vi "Teleop.vi"(10 "Match Info":T2={"Autonomous Elapsed Seconds"=0.0, "TeleOp Elapsed Seconds"=0.0, "Disabled Elapsed Seconds"=0.0, "Visited Autonomous"=FALSE, "Visited TeleOp"=FALSE, "Visited Disabled"=FALSE, "Autonomous Settings"={"Autonomous Style"=enum."Independent", "VI Refnum"=refnum}}, 11 "Call Context":T3) -> ()   [LabVIEW 2023]
doc: "This VI is called for each TeleOp packet received from the DS where the robot is not disabled. It is often used to read from the joysticks and update I/O or to update setpoints for timed control loops. It should complete and return within 20 milliseconds or it may miss DS packets."
uses:
  <vilib>/Rock Robotics/WPI/DriverStation/WPI_DriverStationDerivedRobotMode.ctl
  <vilib>/Rock Robotics/WPI/DriverStation/WPI_DriverStationMatch Info.ctl
  <vilib>/Rock Robotics/WPI/Solenoid/WPI_SolenoidValue.ctl
  <vilib>/Rock Robotics/WPI/ThirdParty/REV Robotics/REVLib/Typedef/Spark MAX Control Type.ctl
  <vilib>/Rock Robotics/Network Tables/NT Read Boolean.vi
  <vilib>/Rock Robotics/Network Tables/NT Read Number.vi
  <vilib>/Rock Robotics/WPI/Solenoid/WPI_SolenoidSetEnum.vi
  <vilib>/Rock Robotics/WPI/Solenoid/WPI_SolenoidGetEnum.vi
panel:
  in  "FIRE!":bool
  in  "spin up SHOOTER":bool
  in  "set motors to ZERO":bool
  out "NOTE DIO":bool
  out "Hard Limit Fwd 2":bool
  out "Hard Limit Rev 2":bool
  out "Hard Limit Fwd":bool
  out "Hard Limit Rev":bool
  out "Value 2":T1
  out "Value":T1
  in  "LOCK?":bool=TRUE
  in  "FLAP?":bool=TRUE
  in  "RIGHT":dbl(slide) scale=-1.0..1.0
  in  "LEFT":dbl(slide) scale=-1.0..1.0
  in  "SHOOTER":dbl(slide) scale=-1.0..1.0
  in  "INTAKE":dbl(slide) scale=-1.0..1.0
  in  "LOADER":dbl(slide) scale=-1.0..1.0
  out "Sample Slider 0":dbl(slide) scale=0.0..5.0
  out "Sample Boolean 1":bool
  out "Sample Boolean 0":bool
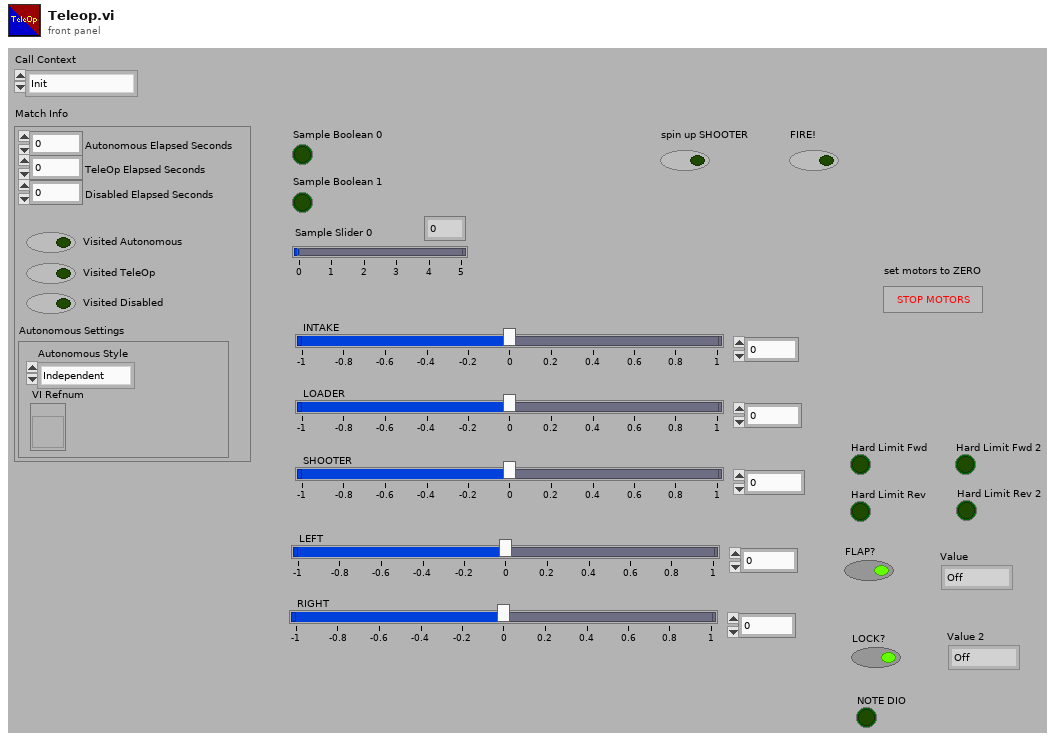
[diagram p1: front panel]
types:
  T1 = typedef "WPI_SolenoidValue.ctl" = enum16{"Off", "On", "Forward", "Reverse"}
  T2 = typedef "WPI_DriverStationMatch Info.ctl" = cluster{"Autonomous Elapsed Seconds":dbl, "TeleOp Elapsed Seconds":dbl, "Disabled Elapsed Seconds":dbl, "Visited Autonomous":bool, "Visited TeleOp":bool, "Visited Disabled":bool, "Autonomous Settings":cluster{"Autonomous Style":enum16{"Iterative", "Independent"}, "VI Refnum":refnum<vi>}}
  T3 = typedef "WPI_DriverStationDerivedRobotMode.ctl" = enum16{"Init", "Execute", "Stop"}
  T4 = typedef "Spark MAX Control Type.ctl" = enum16{"Percent VBus", "Voltage", "Velocity", "Position", "Smart Motion", "Current", "Smart Velocity"}
  T5 = typedef "WPI_MotorControlDeviceRef.ctl" = cluster{"DeviceStatus":errorcluster, "Type":T6, "PWM":cluster{"PWM Channel":T7, "DeadBand":T8}, "CAN":cluster{"Device Number":u8, "SetOutput VI Ref":variant, "GetOutput VI Ref":variant, "Enable VI Ref":variant, "Disable VI Ref":variant, "Data":variant}, "Invert":bool, "DIO PWM":cluster{"PWM \"Enable\" Channel":T7, "DIOChannel":T9, "PWM Rate":dbl}}
  T6 = typedef "WPI_MotorControlType.ctl" = enum16{"PWM", "CAN", "DIO PWM"}
  T7 = typedef "FPGA_DIOPWMChannel.ctl" = enum8{"PWM 0", "PWM 1", "PWM 2", "PWM 3", "PWM 4", "PWM 5", "PWM 6", "PWM 7", "PWM 8", "PWM 9", "PWM MXP 0", "PWM MXP 1", "PWM MXP 2", "PWM MXP 3", "PWM MXP 4", "PWM MXP 5", "PWM MXP 6", "PWM MXP 7", "PWM MXP 8", "PWM MXP 9", "Invalid"}
  T8 = typedef "WPI_PWMDeadband.ctl" = cluster{"Name":string, "maxPositivePwm":i32, "minPositivePwm":i32, "centerPwm":i32, "maxNegativePwm":i32, "minNegativePwm":i32, "angularRange":u16}
  T9 = typedef "FPGA_DIOChannel.ctl" = enum8{"DIO 0", "DIO 1", "DIO 2", "DIO 3", "DIO 4", "DIO 5", "DIO 6", "DIO 7", "DIO 8", "DIO 9", "DIO MXP 0", "DIO MXP 1", "DIO MXP 2", "DIO MXP 3", "DIO MXP 4", "DIO MXP 5", "DIO MXP 6", "DIO MXP 7", "DIO MXP 8", "DIO MXP 9", "DIO MXP 10", "DIO MXP 11", "DIO MXP 12", "DIO MXP 13", "DIO MXP 14", "DIO MXP 15", "SPI Port CS1", "SPI Port CS2", "SPI Port CS3", "SPI Port MISO", "SPI Port MOSI", "Invalid"}
  T10 = typedef "WPI_SolenoidDevRef.ctl" = cluster{"DevStatus":errorcluster, "Pneumatics Control Module":u8, "Forward Solenoid Channel":T11, "Reverse Solenoid Channel":T11}
  T11 = typedef "WPI_SolenoidChannel.ctl" = enum8{"Solenoid 0", "Solenoid 1", "Solenoid 2", "Solenoid 3", "Solenoid 4", "Solenoid 5", "Solenoid 6", "Solenoid 7", "Solenoid 8", "Solenoid 9", "Solenoid 10", "Solenoid 11", "Solenoid 12", "Solenoid 13", "Solenoid 14", "Solenoid 15", "Invalid"}
  T12 = typedef "WPI_DigitalInputDevRef.ctl" = cluster{"DevStatus":errorcluster, "DIO Channel":T9}
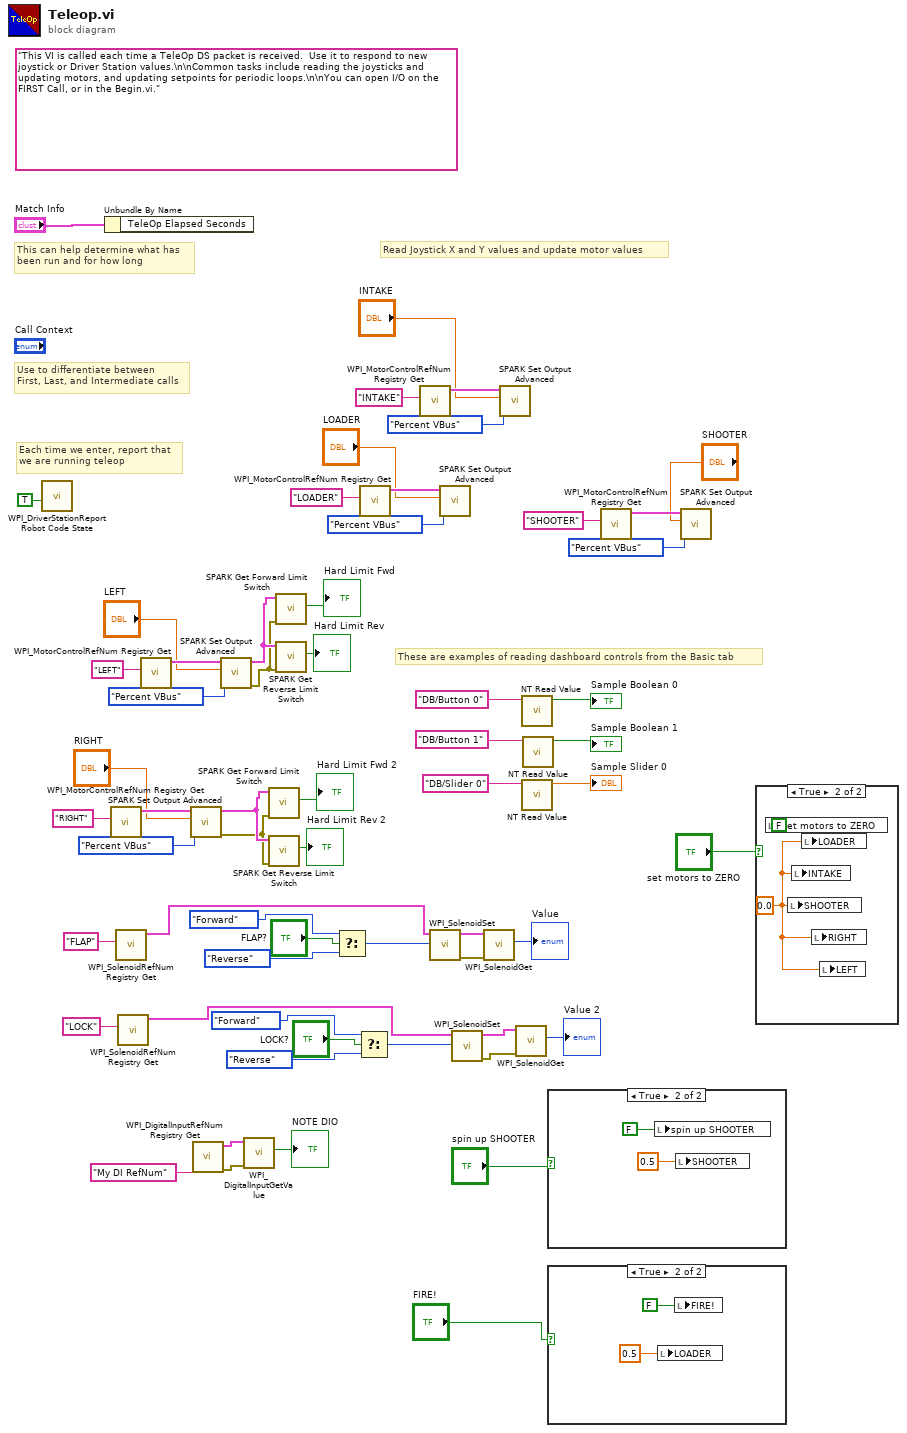
[diagram p0: block diagram]
diagram:
  (unwired) "This VI is called each time a TeleOp DS packet is received.  Use it to respond to new joystick or Driver Station values.\n\nCommon tasks include reading the joysticks and updating motors, and updating setpoints for periodic loops.\n\nYou can open I/O on the FIRST Call, or in the Begin.vi."
  # "These are examples of reading dashboard controls from the Basic tab"
  # "Each time we enter, report that\nwe are running teleop"
  # "Use to differentiate between\nFirst, Last, and Intermediate calls"
  # "This can help determine what has\nbeen run and for how long"
  # "Read Joystick X and Y values and update motor values"
  n1 = call <vilib>:"WPI_DriverStationReport Robot Code State.vi"("TeleOp"=TRUE ("Autonomous")) -> ()  [unwired: 10 in, 1 out]
  n2 = Unbundle By Name("Match Info") -> ()  [unwired: 1 out]
  n3 = call <vilib>:"WPI_MotorControlRefNum Registry Get.vi"("refnum name"="RIGHT") -> ("MotorControlDevRef"=w37:T5)  [unwired: 9 in, 1 out]
  n4 = call <vilib>:"WPI_SolenoidRefNum Registry Get.vi"("refnum name"="FLAP") -> ("SolenoidDevRef"=w22:T10)  [unwired: 9 in, 1 out]
  n5 = call <vilib>:"WPI_SolenoidRefNum Registry Get.vi"("refnum name"="LOCK") -> ("SolenoidDevRef"=w23:T10)  [unwired: 9 in, 1 out]
  n6 = call <vilib>:"WPI_MotorControlRefNum Registry Get.vi"("refnum name"="LEFT") -> ("MotorControlDevRef"=w41:T5)  [unwired: 9 in, 1 out]
  n7 = call <vilib>:"SPARK Set Output Advanced.vi"("Control Mode"=Spark_MAX_Control_Type."Percent VBus", "Setpoint"="RIGHT", "MotorControlDevRef"=w37) -> ("error out"=w8:errorcluster, "MotorControlDevRef"=w9:T5)  [unwired: 7 in]
  n8 = call <vilib>:"WPI_DigitalInputRefNum Registry Get.vi"("refnum name"="My DI RefNum") -> ("error out"=w6:errorcluster, "DigitalInputDevRef"=w5:T12)  [unwired: 9 in]
  n9 = call <vilib>:"SPARK Set Output Advanced.vi"("Control Mode"=Spark_MAX_Control_Type."Percent VBus", "Setpoint"="LEFT", "MotorControlDevRef"=w41) -> ("error out"=w14:errorcluster, "MotorControlDevRef"=w15:T5)  [unwired: 7 in]
  n10 = call <vilib>:"WPI_DigitalInputGetValue.vi"("error in (no error)"=w6, "DigitalInputDevRef"=w5) -> ("Value"=→"NOTE DIO":bool)  [unwired: 7 in, 2 out]
  n11 = call <vilib>:"SPARK Get Forward Limit Switch.vi"("error in (no error)"=w8, "MotorControlDevRef in"=w9) -> ("Hard Limit Fwd"=→"Hard Limit Fwd 2":bool)  [unwired: 6 in, 3 out]
  n12 = call <vilib>:"SPARK Get Reverse Limit Switch.vi"("error in (no error)"=w8, "MotorControlDevRef in"=w9) -> ("Hard Limit Rev"=→"Hard Limit Rev 2":bool)  [unwired: 6 in, 3 out]
  n13 = call <vilib>:"SPARK Get Forward Limit Switch.vi"("error in (no error)"=w14, "MotorControlDevRef in"=w15) -> ("Hard Limit Fwd"=→"Hard Limit Fwd":bool)  [unwired: 6 in, 3 out]
  n14 = call <vilib>:"SPARK Get Reverse Limit Switch.vi"("error in (no error)"=w14, "MotorControlDevRef in"=w15) -> ("Hard Limit Rev"=→"Hard Limit Rev":bool)  [unwired: 6 in, 3 out]
  n15 = Select(t=WPI_SolenoidValue."Forward" ("Value"), s="FLAP?", f=WPI_SolenoidValue."Reverse" ("Value")) -> (s? t:f=w31:T1)
  n16 = Select(t=WPI_SolenoidValue."Forward" ("Value"), s="LOCK?", f=WPI_SolenoidValue."Reverse" ("Value")) -> (s? t:f=w27:T1)
  n17 = call <vilib>:"WPI_MotorControlRefNum Registry Get.vi"("refnum name"="LOADER") -> ("MotorControlDevRef"=w48:T5)  [unwired: 9 in, 1 out]
  n18 = call <vilib>:"WPI_MotorControlRefNum Registry Get.vi"("refnum name"="INTAKE") -> ("MotorControlDevRef"=w52:T5)  [unwired: 9 in, 1 out]
  n19 = call-poly <vilib>:"WPI_SolenoidSet.vi"("Value"=w31, "SolenoidDevRef"=w22) -> ("error out"=w21:errorcluster, "SolenoidDevRef"=w20:T10)  [unwired: 8 in]
  n20 = call <vilib>:"SPARK Set Output Advanced.vi"("Control Mode"=Spark_MAX_Control_Type."Percent VBus", "Setpoint"="LOADER", "MotorControlDevRef"=w48) -> ()  [unwired: 7 in, 2 out]
  n21 = call-poly <vilib>:"WPI_SolenoidSet.vi"("Value"=w27, "SolenoidDevRef"=w23) -> ("error out"=w18:errorcluster, "SolenoidDevRef"=w17:T10)  [unwired: 8 in]
  n22 = call-poly <vilib>:"WPI_SolenoidGet.vi"("error in (no error)"=w21, "SolenoidDevRef"=w20) -> ("Value"=→"Value":T1)  [unwired: 7 in, 2 out]
  n23 = call <vilib>:"SPARK Set Output Advanced.vi"("Control Mode"=Spark_MAX_Control_Type."Percent VBus", "Setpoint"="INTAKE", "MotorControlDevRef"=w52) -> ()  [unwired: 7 in, 2 out]
  n24 = call-poly <vilib>:"WPI_SolenoidGet.vi"("error in (no error)"=w18, "SolenoidDevRef"=w17) -> ("Value"=→"Value 2":T1)  [unwired: 7 in, 2 out]
  n25 = call-poly <vilib>:"NT Read Value.vi"("name"="DB/Button 0" ("refnum name")) -> ("value"=→"Sample Boolean 0":bool)  [unwired: 8 in, 2 out]
  n26 = call-poly <vilib>:"NT Read Value.vi"("name"="DB/Slider 0" ("refnum name")) -> ("value"=→"Sample Slider 0":dbl)  [unwired: 8 in, 2 out]
  n27 = call-poly <vilib>:"NT Read Value.vi"("name"="DB/Button 1" ("refnum name")) -> ("value"=→"Sample Boolean 1":bool)  [unwired: 8 in, 2 out]
  n28 = case shown="True" "spin up SHOOTER" {
    frame False {
    }
    frame True {
      n29 = local write "spin up SHOOTER"(FALSE ("spin up SHOOTER")) -> ()
      n30 = local write "SHOOTER"(0.5 ("SHOOTER")) -> ()
    }
  }
  n31 = case shown="True" "FIRE!" {
    frame False {
    }
    frame True {
      n32 = local write "LOADER"(0.5 ("LOADER")) -> ()
      n33 = local write "FIRE!"(FALSE ("FIRE!")) -> ()
    }
  }
  n34 = call <vilib>:"WPI_MotorControlRefNum Registry Get.vi"("refnum name"="SHOOTER") -> ("MotorControlDevRef"=w44:T5)  [unwired: 9 in, 1 out]
  n35 = call <vilib>:"SPARK Set Output Advanced.vi"("Control Mode"=Spark_MAX_Control_Type."Percent VBus", "Setpoint"="SHOOTER", "MotorControlDevRef"=w44) -> ()  [unwired: 7 in, 2 out]
  n36 = case shown="True" "set motors to ZERO" {
    frame False {
    }
    frame True {
      w66 = 0.0 ("SHOOTER")
      n37 = local write "set motors to ZERO"(FALSE ("stop")) -> ()
      n38 = local write "SHOOTER"(w66) -> ()
      n39 = local write "INTAKE"(w66) -> ()
      n40 = local write "LOADER"(w66) -> ()
      n41 = local write "RIGHT"(w66) -> ()
      n42 = local write "LEFT"(w66) -> ()
    }
  }
